vi "Obtain Message Queue.vi"(8 "error in (no error)":errorcluster caption="에러 입력(에러 없음)") -> (0 "error out":errorcluster caption="에러 출력", 3 "Message Queue":refnum<queue> caption="메시지 큐")   [LabVIEW 2018, in "Message Queue.lvlib"]
doc: "메시지 클러스터 데이터 타입이 포함된 큐를 생성합니다."
uses:
  Message Queue.lvlib
  Message Cluster.ctl
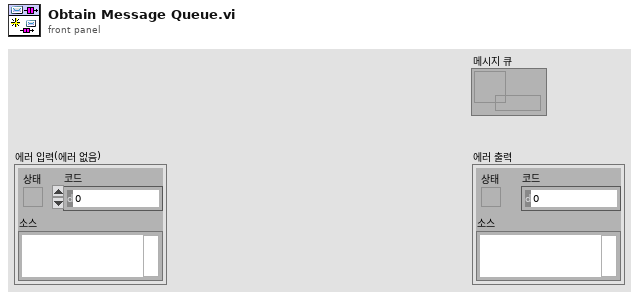
[diagram p1: front panel]
types:
  T1 = typedef "Message Queue.lvlib/Message Cluster.ctl" = cluster{"Message":string, "Message Data":variant}
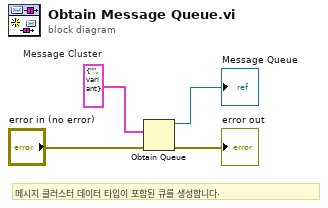
[diagram p0: block diagram]
diagram:
  w4 = T1 {"Message"="", "Message Data"=variant}  # Message Cluster
  # "메시지 클러스터 데이터 타입이 포함된 큐를 생성합니다."
  n1 = Obtain Queue(element data type=w4, error in (no error)="error in (no error)") -> (queue out=→"Message Queue":refnum<queue>, error out=→"error out":errorcluster)  [unwired: 3 in, 1 out]
